vi "Get All Running Measurement Queues.vi"(8 "error in (no error)":errorcluster, 11 "Mag Lab Measure Controller in":refnum<class "Mag Lab Measure Controller.lvclass">) -> (0 "error out":errorcluster, 2 "Array of Measurement Queues":refnum<class "Message Enqueuer.lvclass">[](array[class]), 3 "Mag Lab Measure Controller out":refnum<class "Mag Lab Measure Controller.lvclass">)   [LabVIEW 2015, in "Mag Lab Measure Controller.lvclass"]
uses:
  Mag Lab Measure Controller.lvclass
  <vilib>/ActorFramework/Message Enqueuer/Message Enqueuer.lvclass
  Mag Lab Measure Controller.lvclass/Mag Lab Measure Controller.ctl
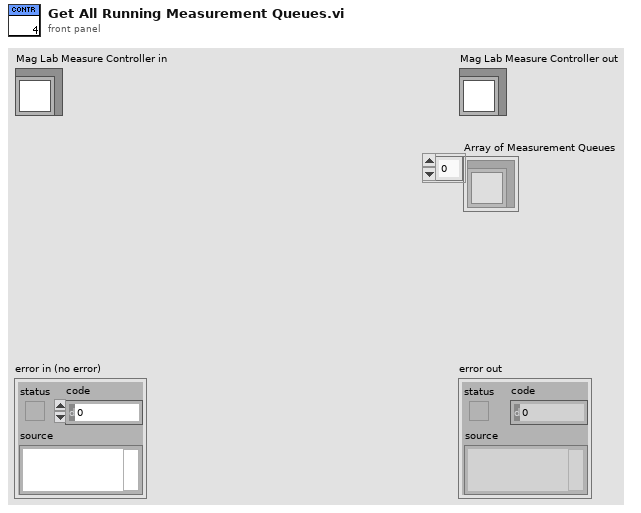
[diagram p1: front panel]
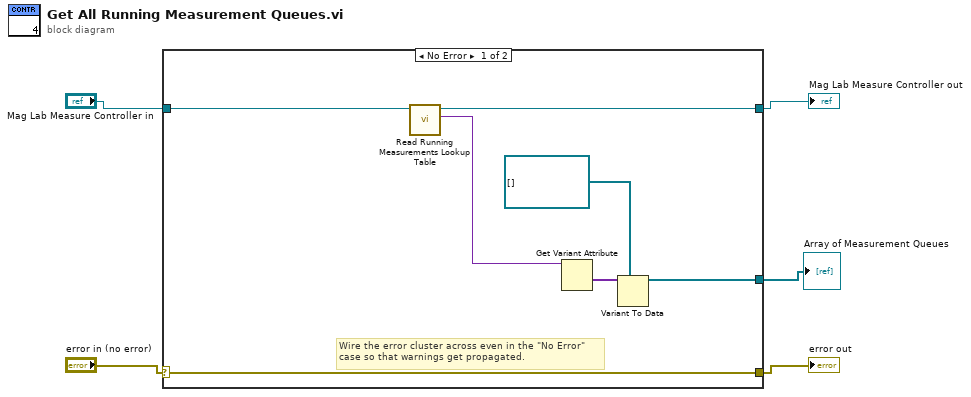
[diagram p0: block diagram]
diagram:
  n1 = case shown="No Error" "error in (no error)" {
    selector: "error in (no error)" -> [w12 w14]
    tunnel: [w12 w14] -> w4
    tunnel: [w8 w13] -> w5
    tunnel: "Mag Lab Measure Controller in" -> [w9 w13]
    tunnel: [w7 _] -> w1
    frame No Error {
      # "Wire the error cluster across even in the \"No Error\"\ncase so that warnings get propagated."
      n2 = call "Read Running Measurements Lookup Table.vi"("Mag Lab Measure Controller in"=w9) -> ("Running Measurements Queue Lookup Table"=w11:variant, "Mag Lab Measure Controller out"=w8:refnum<class "Mag Lab Measure Controller.lvclass">)  [unwired: 8 in, 1 out]
      n3 = Get Variant Attribute(Variant=w11) -> (values=w10:variant[])  [unwired: 3 in, 3 out]
      n4 = Variant To Data(type=refnum<class "Message Enqueuer.lvclass">[] [], Variant=w10) -> (data=w7:refnum<class "Message Enqueuer.lvclass">[])  [unwired: 1 in, 1 out]
    }
    frame Error {
    }
  }
  "error out" <- w4
  "Mag Lab Measure Controller out" <- w5
  "Array of Measurement Queues" <- w1
